vi "convert tcp data (host command).vi"(8 "error in":errorcluster, 11 "TCP_DATA":string) -> (0 "error out":errorcluster, 1 "value":string, 2 "ChNo":u16, 3 "command":T1 items=["NO_Action", "start", "pause", "resum", "stop", "config", "System_constant", "7", "DAQ_init", "DAQ_config", "DAQ_start", "DAQ_read", "DAQ_stop", "DAQ_contrl", "14", "15", "16", "17", "18", "19", "Zsf_open", "Zsf_close", "Wkf_control", "Pump_switch", "dcf_switch", "JRQ_switch"])   [LabVIEW 2011]
uses:
  Ctrls/command.ctl
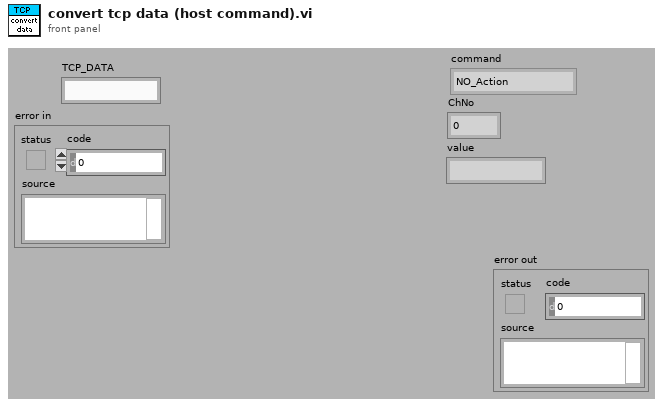
[diagram p1: front panel]
types:
  T1 = typedef "command.ctl" = u16
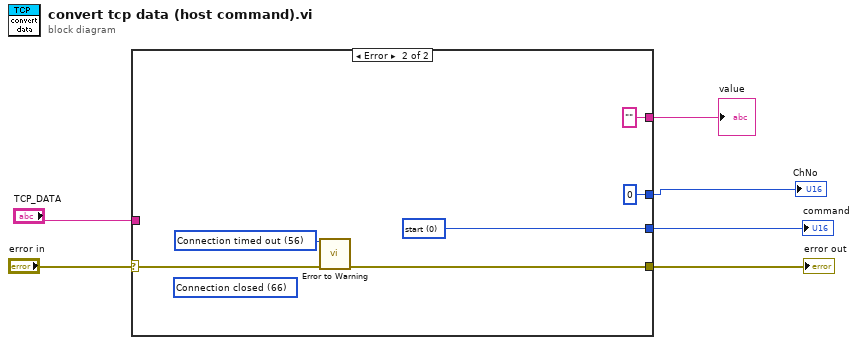
[diagram p0: block diagram]
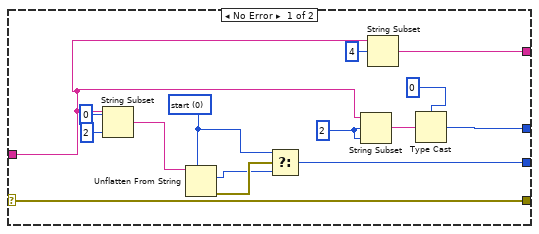
[diagram p2: hidden frame]
diagram:
  n1 = case shown="Error" "error in" {
    selector: "error in" -> [w21 w25]
    tunnel: [w21 w24] -> w6
    tunnel: [w18 w27] -> w5
    tunnel: "TCP_DATA" -> [w9 _]
    tunnel: [w10 u16 0] -> w2
    tunnel: [w7 "" ("TCP_DATA")] -> w1
    frame No Error {
      w13 = 2 ("offset (0)")
      w19 = T1 0 items=["start", "pause", "resum", "stop"] ("command")
      n2 = String Subset(string=w9, offset (0)=0, length (rest)=2 ("length (rest)")) -> (substring=w15:string)
      n3 = Unflatten From String(type=w19, binary string=w15) -> (value=w17:T1, error out=w20:errorcluster)  [unwired: 3 in, 1 out]
      n4 = Select(t=w19, s=w20, f=w17) -> (s? t:f=w18:T1)
      n5 = String Subset(string=w9, offset (0)=w13, length (rest)=w13) -> (substring=w12:string)
      n6 = String Subset(string=w9, offset (0)=4) -> (substring=w7:string)  [unwired: 1 in]
      n7 = Type Cast(type=u16 0, x=w12) -> (*(type *) &x=w10:u16)
    }
    frame Error {
      w27 = T1 0 items=["start", "pause", "resum", "stop"] ("command")
      (unwired) 66 items=["No Error", "Argument Error", "Memory Full", "Out of Zone", "End of File", "File Already Open", "Generic File IO Error", "File Not Found", "File Permission Error", "Disk Full", "Duplicate Path", "Too Many Files Open", "Not Enabled", "Resource File Not Found", "Cannot Add Resource", "Resource Not Found", "Image Not Found", "Image Memory Error", "Pen Does Not Exist", "Config Bad Type", "Config Token Not Found", "Config Parse Error", "Config Memory Error", "Bad External Code Format", "Bad External Code Offset", "External Code Not Present", "Null Window", "Destroy Window Mixup", "Null Menu", "Print Aborted", "Bad Print Record", "Print Driver Error", "Windows Error During Print", "Memory Error During Print", "Print Dialog Error", "Generic Print Error", "Invalid Device Refnum", "Device Not Found", "Device Parameter Error", "Device Unit Error", "Can't Open Device", "Device Call Aborted", "Generic Error", "Cancelled By User", "Object ID Too Low", "Object ID Too High", "Object Not In Heap", "Unknown Heap", "Bad DefProc ID", "DefProc Not In Table", "Message Out Of Range", "Null Method", "Unknown Message", "Manager Call Not Supported", "Bad address", "Connection In progress", "Connection timed out", "Connection is already in progress", "Network attribute not supported", "Network error", "Address in use", "System out of memory", "Connection aborted", "Connection refused", "Connection is not connected", "Connection is already connected", "Connection closed", "Initialize error (interapplication manager)", "Bad occurrence", "Wait on unbound occurrence handler", "Occurrence queue overflow", "Bad path", "Semaphore not signaled", "Unrecognized type (interapplication manager)"] ("2nd Error to Convert")
      w26 = 56 items=["No Error", "Argument Error", "Memory Full", "Out of Zone", "End of File", "File Already Open", "Generic File IO Error", "File Not Found", "File Permission Error", "Disk Full", "Duplicate Path", "Too Many Files Open", "Not Enabled", "Resource File Not Found", "Cannot Add Resource", "Resource Not Found", "Image Not Found", "Image Memory Error", "Pen Does Not Exist", "Config Bad Type", "Config Token Not Found", "Config Parse Error", "Config Memory Error", "Bad External Code Format", "Bad External Code Offset", "External Code Not Present", "Null Window", "Destroy Window Mixup", "Null Menu", "Print Aborted", "Bad Print Record", "Print Driver Error", "Windows Error During Print", "Memory Error During Print", "Print Dialog Error", "Generic Print Error", "Invalid Device Refnum", "Device Not Found", "Device Parameter Error", "Device Unit Error", "Can't Open Device", "Device Call Aborted", "Generic Error", "Cancelled By User", "Object ID Too Low", "Object ID Too High", "Object Not In Heap", "Unknown Heap", "Bad DefProc ID", "DefProc Not In Table", "Message Out Of Range", "Null Method", "Unknown Message", "Manager Call Not Supported", "Bad address", "Connection In progress", "Connection timed out", "Connection is already in progress", "Network attribute not supported", "Network error", "Address in use", "System out of memory", "Connection aborted", "Connection refused", "Connection is not connected", "Connection is already connected", "Connection closed", "Initialize error (interapplication manager)", "Bad occurrence", "Wait on unbound occurrence handler", "Occurrence queue overflow", "Bad path", "Semaphore not signaled", "Unrecognized type (interapplication manager)"] ("1st Error to Convert")
      n8 = call <vilib>:"Error to Warning.vi"("1st Error to Convert"=w26, "error in"=w25) -> ("warning out"=w24:errorcluster)  [unwired: 13 in]
    }
  }
  "command" <- w5
  "error out" <- w6
  "ChNo" <- w2
  "value" <- w1
